vi "test Copy To Smaller Destination.vi"(8 "error in (no error)":errorcluster, 11 "TestCase in":refnum<class "Data Manipulation Tests.lvclass">) -> (0 "error out":errorcluster, 3 "TestCase out":refnum<class "Data Manipulation Tests.lvclass">)   [LabVIEW 2017, in "Pointer Tests.lvlib" / "Data Manipulation Tests.lvclass"]
uses:
  Data Manipulation Tests.lvclass
  Source/Classes/Pointer/Pointer.lvclass/Pointer.ctl
  Source/Classes/Pointer/Public/New/New (4B).vi
  Source/Classes/Pointer/Public/Write/Write (1D I32).vi
  Source/Classes/Pointer/Public/New/New (2B).vi
  Source/Classes/Pointer/Public/Read/Read (1D I32).vi
  Source/Classes/Pointer/Private/Allocate.vi
  Source/Classes/Pointer/Public/Write (No Check)/Write (No Check 1D I32).vi
  Source/Classes/Pointer/Protected/Parameter Checking/Check Null Pointer.vi
  Source/Classes/Pointer/Protected/Parameter Checking/Check Subset (Power of 2).vi
  Source/Classes/Pointer/API/Accessors/Get Size.vi
  Source/Classes/Pointer/Public/Copy (No Check).vi
  Source/Classes/Pointer/Protected/Parameter Checking/Check Subset.vi
  Source/Classes/Pointer/Public/Read (No Check)/Read (No Check 1D I32).vi
  Source/Classes/Pointer/Private/Deallocate.vi
  Source/Classes/Pointer/API/Accessors/Set Address.vi
  Source/Classes/Pointer/API/Accessors/Set Size.vi
  Source/Classes/Pointer/Private/Set Internal.vi
  Source/Classes/Pointer/API/Accessors/Get Address.vi
  Source/Classes/Pointer/Protected/Errors.vi
  Source/Classes/Pointer/Protected/Error VIs/Null Pointer.vi
  Source/Classes/Pointer/Protected/Error VIs/Out of Bounds.vi
  Source/Classes/Pointer/Private/Count to Size.vi
  Source/Classes/Pointer/Protected/Get Internal.vi
  Source/Classes/Pointer/Protected/Error VIs/Zone.vi
  Source/Classes/Pointer/Protected/Error Building/Create Error.vi
  Source/VIs/Write String into Source.vi
  Source/Classes/Pointer/Protected/Error Building/Write Pointer Size.vi
  Source/VIs/Write Number into Source.vi
  Source/VIs/VIs for Poly/Write U64 into Source.vi
  Source/Constants/Constants.vi
  Source/Constants/Library Name.vi
  Source/Classes/Pointer/Protected/Error Building/Get Error Info.vi
  Source/VIs/Create Error Cluster.vi
  Source/VIs/VIs for Poly/Create Error Cluster (256B).vi
  Source/VIs/Set Error Status.vi
  Source/VIs/Set Error Code.vi
  Source/VIs/Set Error Source.vi
  Source/Classes/Pointer/Pointer.lvclass
  <vilib>/addons/_JKI Toolkits/VI Tester/TestCase.llb/TestCase.lvclass
  C:/Program Files (x86)/National Instruments/LabVIEW 2017/vi.lib/addons/_JKI Toolkits/VI Tester/TestCase.llb/TestCase.lvclass
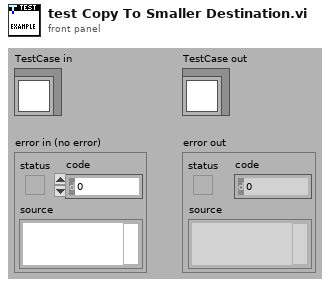
[diagram p1: front panel]
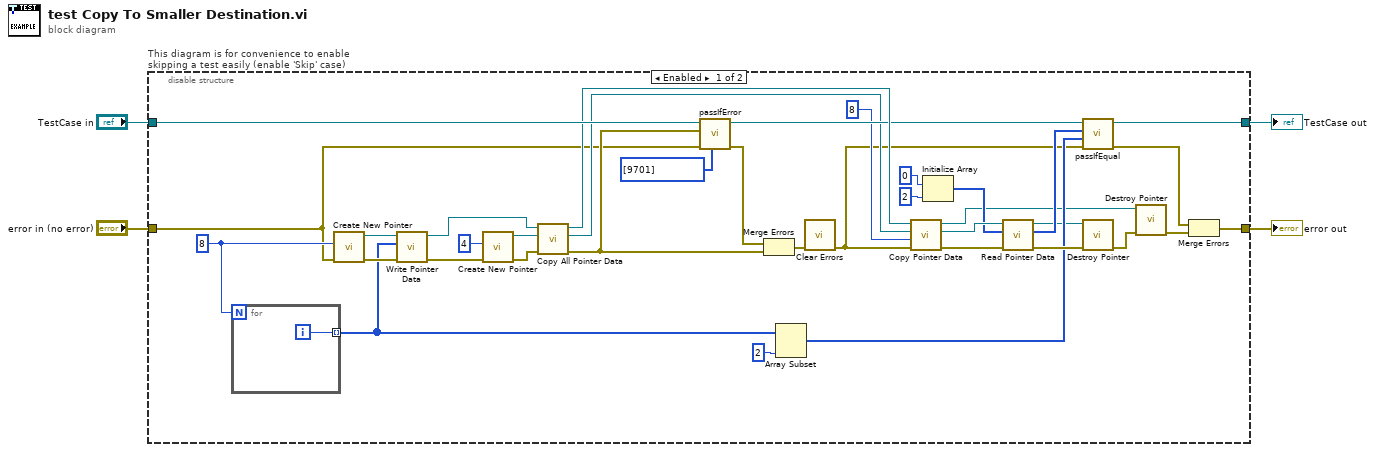
[diagram p0: block diagram]
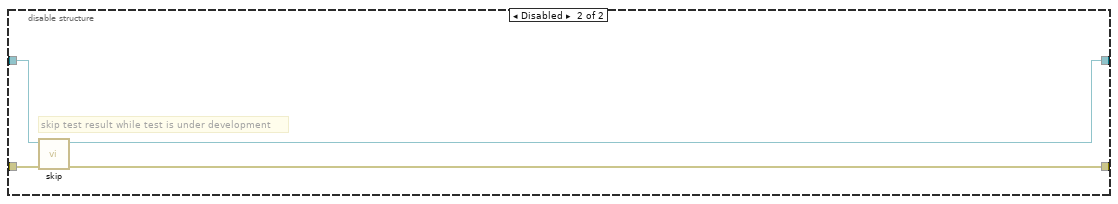
[diagram p2: hidden frame]
diagram:
  n1 = disable-structure "This diagram is for convenience to enable skipping a test easily (enable 'Skip' case)" shown="Enabled" {
    disable-tunnel: "TestCase in" -> [w37 w45]
    disable-tunnel: [w21 w43] -> w1
    disable-tunnel: [w33 w44] -> w3
    disable-tunnel: "error in (no error)" -> [w6 w42]
    frame Enabled {
      w25 = u64 8 ("count (1)")
      n2 = for {
        N: w25 -> [_]
        tunnel: [w41] -> w16 mode=indexing
        i -> [w41]
      }
      n3 = call-poly "Create New Pointer.vi"("error in (no error)"=w6, "count (1)"=w25) -> ("error out"=w36:errorcluster, "Pointer"=w40:refnum<class "Pointer.lvclass">)  [unwired: 8 in]
      n4 = call-poly "Write Pointer Data.vi"("error in (no error)"=w36, "buffer in"=w16, "Pointer in"=w40) -> ("error out"=w35:errorcluster, "Pointer out"=w39:refnum<class "Pointer.lvclass">)  [unwired: 5 in, 2 out]
      n5 = call-poly "Create New Pointer.vi"("error in (no error)"=w35, "count (1)"=u64 4) -> ("error out"=w34:errorcluster, "Pointer"=w38:refnum<class "Pointer.lvclass">)  [unwired: 8 in]
      n6 = call "Copy All Pointer Data.vi"("error in (no error)"=w34, "dst Pointer in"=w38, "src Pointer in"=w39) -> ("error out"=w31:errorcluster, "dst Pointer out"=w17:refnum<class "Pointer.lvclass">, "src Pointer out"=w29:refnum<class "Pointer.lvclass">)  [unwired: 6 in]
      n7 = call-dynamic "passIfError.vi"("passing error codes (default = any error code)"=i32[] [9701], "error in (no error)"=w6, "error"=w31, "TestCase in"=w37) -> ("error out"=w8:errorcluster, "TestCase out"=w22:refnum<class "Data Manipulation Tests.lvclass">)  [unwired: 6 in]
      n8 = Merge Errors(w8, w31) -> (w7:errorcluster)
      n9 = Array Subset(array=w16, length=2) -> (w14:i32[])  [unwired: 1 in]
      n10 = call <vilib>:"Clear Errors.vi"("error in (no error)"=w7) -> ("error out"=w5:errorcluster)  [unwired: 5 in, 1 out]
      n11 = call "Copy Pointer Data.vi"("error in (no error)"=w5, "bytes to copy"=u64 8, "dst Pointer in"=w17, "src Pointer in"=w29) -> ("error out"=w30:errorcluster, "dst Pointer out"=w27:refnum<class "Pointer.lvclass">, "src Pointer out"=w9:refnum<class "Pointer.lvclass">)  [unwired: 4 in, 1 out]
      n12 = Initialize Array(0 ("Numeric"), 2 ("dimension size")) -> (w24:i32[])
      n13 = call-poly "Read Pointer Data.vi"("error in (no error)"=w30, "buffer in"=w24, "Pointer in"=w27) -> ("error out"=w28:errorcluster, "buffer out"=w20:i32[], "Pointer out"=w11:refnum<class "Pointer.lvclass">)  [unwired: 5 in, 1 out]
      n14 = call-dynamic "passIfEqual.vi"("error in (no error)"=w5, "y"=w14, "x"=w20, "TestCase in"=w22) -> ("error out"=w23:errorcluster, "TestCase out"=w21:refnum<class "Data Manipulation Tests.lvclass">)  [unwired: 6 in]
      n15 = call "Destroy Pointer.vi"("error in (no error)"=w28, "Pointer in"=w11) -> ("error out"=w12:errorcluster)  [unwired: 8 in, 1 out]
      n16 = call "Destroy Pointer.vi"("error in (no error)"=w12, "Pointer in"=w9) -> ("error out"=w10:errorcluster)  [unwired: 8 in, 1 out]
      n17 = Merge Errors(w23, w10) -> (w33:errorcluster)
    }
    frame Disabled {
      # "skip test result while test is under development"
      n18 = call <vilib>:"skip.vi"("error in (no error)"=w42, "TestCase in"=w45) -> ("error out"=w44:errorcluster, "TestCase out"=w43:refnum<class "Data Manipulation Tests.lvclass">)  [unwired: 8 in]
    }
  }
  "error out" <- w3
  "TestCase out" <- w1
